vi "VCS Get Protocol Stack Settings.vi"(8 "error in (no error)":errorcluster, 11 "keyHandle in":u32) -> (0 "error out":errorcluster, 2 "settings":cluster{"baudrate":u32, "timeout":u32}, 3 "keyHandle out":u32)   [LabVIEW 2010]
doc: "<B>VCS Get Protocol Stack Settings</B> reads the communication parameters."
uses:
  Resources/EposCmd.dll
  Resources/EposCmd64.dll
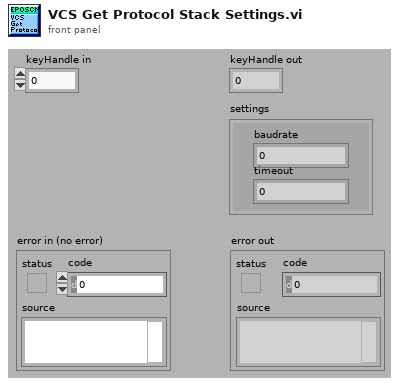
[diagram p1: front panel]
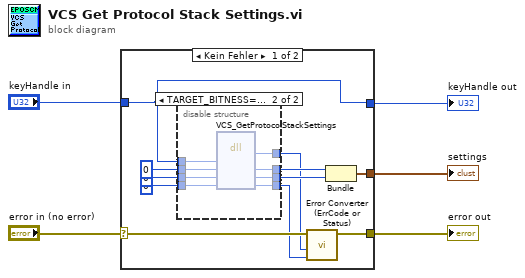
[diagram p0: block diagram]
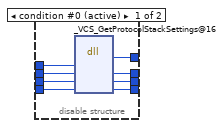
[diagram p2: hidden frame]
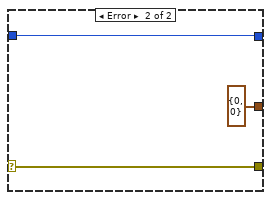
[diagram p3: hidden frame]
diagram:
  n1 = case shown="Kein Fehler" "error in (no error)" {
    selector: "error in (no error)" -> [w16 w35]
    tunnel: [w15 w35] -> w4
    tunnel: [w10 cluster{"pBaudrate":u32, "pTimeout":u32} {"pBaudrate"=0, "pTimeout"=0}] -> w3
    tunnel: "keyHandle in" -> [w7 w33]
    tunnel: [w7 w33] -> w1
    frame No Error {
      n2 = disable-structure shown="TARGET_BITNESS==64" {
        disable-tunnel: [w24 w32] -> w14
        disable-tunnel: u32 0 ("pBaudrate") -> [w23 w31]
        disable-tunnel: [w22 w30] -> w12
        disable-tunnel: [w21 w29] -> w11
        disable-tunnel: u32 0 ("pTimeout") -> [w20 w28]
        disable-tunnel: u32 0 ("pErrorCode") -> [w19 w27]
        disable-tunnel: w7 -> [w18 w26]
        disable-tunnel: [w17 w25] -> w6
        frame condition #0 (active) {
          n3 = dll-call lib="C:/Sources/LabView/maxon EPOS/Resources/EposCmd.*" fn="_VCS_GetProtocolStackSettings@16"("KeyHandle"=w18, "pBaudrate"=w23, "pTimeout"=w20, "pErrorCode"=w19) -> (w17:i32, "pBaudrate"=w22:u32, "pTimeout"=w21:u32, "pErrorCode"=w24:u32)  [unwired: 4 in, 2 out]
        }
        frame condition #1 {
          n4 = dll-call lib="C:/setup/Resources/EposCmd64.dll" fn="VCS_GetProtocolStackSettings" ("EposCmd.dll:_VCS_GetProtocolStackSettings@16")("KeyHandle"=w26, "pBaudrate"=w31, "pTimeout"=w28, "pErrorCode"=w27) -> ("return type"=w25:i32, "pBaudrate"=w30:u32, "pTimeout"=w29:u32, "pErrorCode"=w32:u32)  [unwired: 4 in, 2 out]
        }
      }
      n5 = call "Error Converter (ErrCode or Status).vi"("error code"=w14, "return type"=w6, "error in (no error)"=w16) -> ("error out"=w15:errorcluster)  [unwired: 7 in]
      n6 = Bundle("pBaudrate"=w12, "pTimeout"=w11) -> (w10:cluster{"pBaudrate":u32, "pTimeout":u32})  [unwired: 1 in]
    }
    frame Error {
    }
  }
  "error out" <- w4
  "settings" <- w3
  "keyHandle out" <- w1
